vi "ExpandEnvironmentStrings_IWsh.vi"(6 "error in (no error)":errorcluster, 9 "String w/ \nEnvironment Variable(s)":string) -> (0 "error out":errorcluster, 2 "EnvVar(s) Found":bool, 3 "Expanded String":string)   [LabVIEW 2013]
doc: "This VI allows the user to access environmental variables on the system. Either use the enum for the MMCD standard environmental variables or input one manual. Manual input overrides the enum."
panel:
  in  "IWshRuntimeLibrary.IWshShell2":refnum<k7>
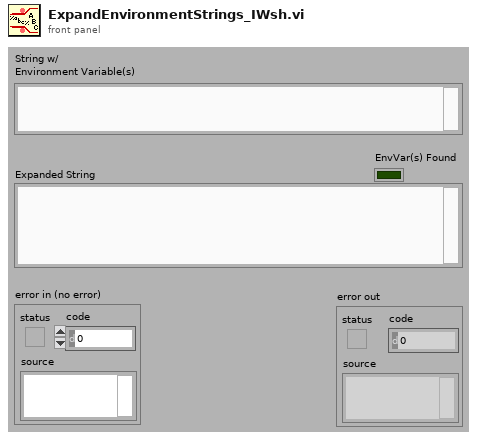
[diagram p1: front panel]
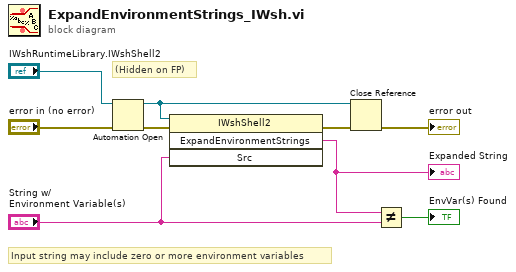
[diagram p0: block diagram]
diagram:
  # "Input string may include zero or more environment variables"
  # "(Hidden on FP)"
  n1 = Automation Open(error in (no error)="error in (no error)", Automation Refnum="IWshRuntimeLibrary.IWshShell2") -> (Automation Refnum=w6:refnum<k7>, error out=w2:errorcluster)  [unwired: 2 in]
  n2 = invoke class="IWshShell2" method="ExpandEnvironmentStrings"(reference=w6, error in=w2, "Src"="String w/ \nEnvironment Variable(s)") -> (error out=w7:errorcluster, "ExpandEnvironmentStrings"=w4:string)  [unwired: 1 in, 2 out]
  "Expanded String" <- w4
  n3 = Close Reference(reference=w6, error in (no error)=w7) -> (error out=→"error out":errorcluster)
  n4 = Not Equal?(x=w4, y="String w/ \nEnvironment Variable(s)") -> (x != y?=→"EnvVar(s) Found":bool)
